vi "CloseFont.vi"(8 "No Error":errorcluster, 11 "Font [TTF_Font *]":T1 format="%.0x") -> (0 "error out":errorcluster)   [LabVIEW 2026, in "SDL3.lvlib" / "TTF.lvlib"]
doc: "<B>Summary</B>\nDispose of a previously-created font.\n\n<B>Remarks</B>\nCall this when done with a font. This function will free any resources associated with it. It is safe to call this function on NULL, for example on the result of a failed call to <B>TTF_OpenFont()</B>.\n\nThe font is not valid after being passed to this function. String pointers from functions that return information on this font, such as <B>TTF_GetFontFamilyName()</B> and <B>TTF_GetFontStyleName()</B>, are no longer valid after this call, as well."
uses:
  TTF.lvlib
  Lib/SDL3_ttf.dll
  TTF_Font--pointer.ctl
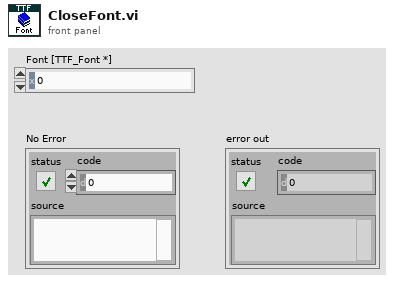
[diagram p1: front panel]
types:
  T1 = typedef "SDL3.lvlib/TTF.lvlib/TTF_Font--pointer.ctl" = i64
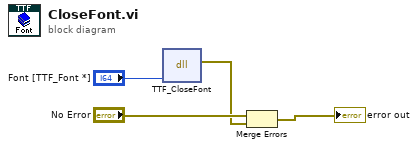
[diagram p0: block diagram]
diagram:
  n1 = dll-call lib="C:/Users/saukko/Dev/LV-SDL3/Sources/SDL3/Lib/SDL3_ttf.*" fn="TTF_CloseFont"("font"="Font [TTF_Font *]") -> (error out=w1:errorcluster)  [unwired: 5 in, 1 out]
  n2 = Merge Errors("No Error", w1) -> (→"error out":errorcluster)
